vi "Right Click Menu Configuration.vi"(7 "MCListbox Refnum":refnum<vi>, 10 "Coords":T1, 11 "MenuRef":refnum<k9>) -> (0 "error out":errorcluster)   [LabVIEW 2016, in "Assert API Components.lvlib" / "Assert Display.lvlib" / "Main Display.lvlib" / "Main Display.lvclass"]
uses:
  Main Display.lvclass
  <vilib>/Utility/miscctls.llb/LVPoint32TypeDef.ctl
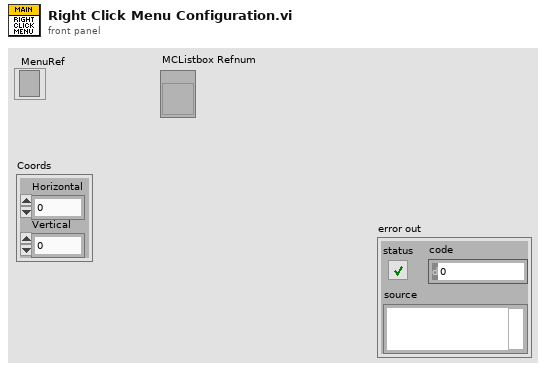
[diagram p1: front panel]
types:
  T1 = typedef "LVPoint32TypeDef.ctl" = cluster{"Horizontal":i32, "Vertical":i32}
  T2 = typedef "LVRowAndColumnTypeDef.ctl" = cluster{"Row":i32, "Column":i32}
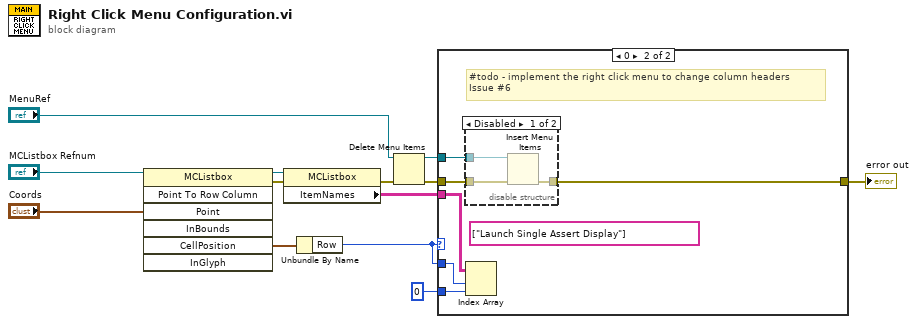
[diagram p0: block diagram]
diagram:
  n1 = invoke class="MCListbox" method="Point To Row Column"(reference="MCListbox Refnum", "Point"="Coords") -> (reference out=w8:refnum<vi>, error out=w4:errorcluster, "CellPosition"=w9:T2)  [unwired: 5 in, 4 out]
  n2 = property class="MCListbox"(reference=w8, error in=w4) -> (error out=w5:errorcluster, "ItemNames"=w7:string[][])  [unwired: 1 out]
  n3 = Unbundle By Name(w9) -> ("Row"=w1:i32)
  n4 = Delete Menu Items(6:w5, 9:"MenuRef") -> (0:w2:errorcluster, 3:w3:refnum<k9>)  [unwired: 2 in]
  n5 = case shown="0" w1 {
    tunnel: [w14 w20] -> w10
    tunnel: w7 -> [_ w19]
    tunnel: w1 -> [_ w18]
    tunnel: 0 ("disabled index (col)") -> [_ w17]
    tunnel: w3 -> [_ w16]
    tunnel: w2 -> [w14 w15]
    frame Default {
    }
    frame 0 {
      (unwired) string[] ["Launch Single Assert Display"] ("item names")
      # "#todo - implement the right click menu to change column headers\nIssue #6"
      n6 = disable-structure shown="Disabled" {
        disable-tunnel: [w23 _] -> w20
        disable-tunnel: w16 -> [w22 _]
        disable-tunnel: w15 -> [w21 _]
        frame Disabled {
          n7 = Insert Menu Items(6:w21, 9:w22) -> (0:w23:errorcluster)  [unwired: 4 in, 2 out]
        }
        frame Enabled {
        }
      }
      n8 = Index Array(array=w19, index (row)=w18, index (col)=w17) -> ()  [unwired: 1 out]
    }
  }
  "error out" <- w10
